vi "Send_Command.vi"(1 "write buffer":string, 2 "VISA resource name":refnum<visa-resource-name>) -> (0 "Command sent":bool)   [LabVIEW 2018]
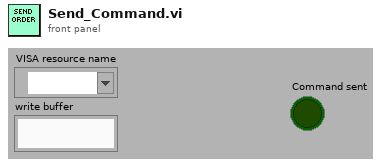
[diagram p1: front panel]
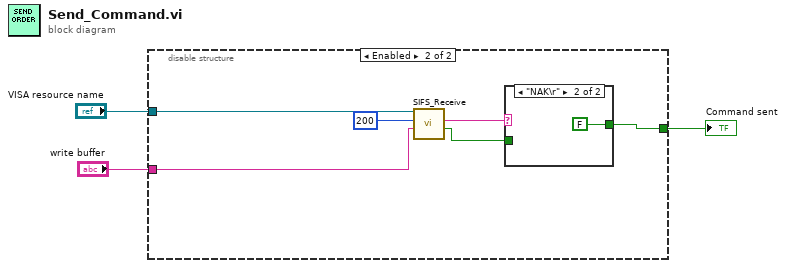
[diagram p0: block diagram]
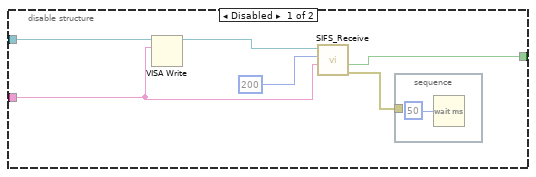
[diagram p2: hidden frame]
diagram:
  n1 = disable-structure shown="Enabled" {
    disable-tunnel: "VISA resource name" -> [w7 w15]
    disable-tunnel: "write buffer" -> [w6 w14]
    disable-tunnel: [w5 w12] -> w1
    frame Disabled {
      n2 = VISA Write(VISA resource name=w7, write buffer=w6) -> (VISA resource name out=w9:refnum<visa-resource-name>)  [unwired: 1 in, 2 out]
      n3 = call "SIFS_Receive.vi"("Command to SIFS"=w6, "wait after tx"=u32 200 ("milliseconds to wait"), "VISA resource name"=w9) -> ("error out"=w4:errorcluster, "cmd sent"=w5:bool)  [unwired: 1 in, 2 out]
      n4 = stacked-sequence {
        tunnel: w4 -> [_]
        frame #0 {
          n5 = Wait (ms)(milliseconds to wait=u32 50) -> ()  [unwired: 1 out]
        }
      }
    }
    frame Enabled {
      n6 = call "SIFS_Receive.vi"("Command to SIFS"=w14, "wait after tx"=u32 200 ("milliseconds to wait"), "VISA resource name"=w15) -> ("cmd sent"=w11:bool, "Response from SIFS"=w13:string)  [unwired: 1 in, 2 out]
      n7 = case shown="\"NAK\\r\"" w13 {
        tunnel: [w17 FALSE] -> w12
        tunnel: w11 -> [w17 _]
        frame "False", Default {
        }
        frame "NAK\r" {
        }
      }
    }
  }
  "Command sent" <- w1
